vi "SYST_SHOR_PATH.vi"(0 "VISA IN":refnum<visa-resource-name>, 1 "Path":string, 5 "error in":errorcluster, 7 "Number":i32) -> (14 "VISA Out":refnum<visa-resource-name>, 19 "error out":errorcluster)   [LabVIEW 2018, in "PNA-X.lvlib"]
doc: "SYSTem:SHORtcut<n>:PATH <string> \n(Read-Write) Defines a Macro (shortcut) by linking a path and file name to the Macro number. To be \nexecuted, the executable file must be put in the PNA at the location indicated by this command. \nParameters \n<n> Numeric. Number of the macro to be stored in the analyzer. If the index \nnumber already exists, the existing macro is replaced with the new macro. \n<string> Full path, file name, and extension, of the existing macro \"executable\" file. \nTo find the number of a macro, either open the Macro Setup dialog and count \nthe line number of the desired macro, or query the titles of all 12 macros for the \ndesired macro title. \nExamples SYST:SHOR1:PATH \"C:\\Program Files\\Agilent\\Network \nAnalyzer\\Documents\\unguideMultiple.vbs\" \nQuery Syntax SYSTem:SHORtcut<n>:PATH? \nDefault Not Applicable"
uses:
  PNA-X.lvlib
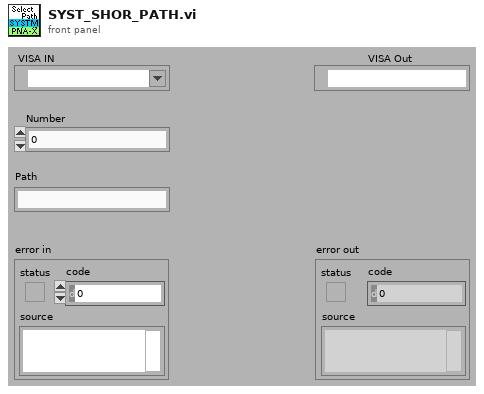
[diagram p1: front panel]
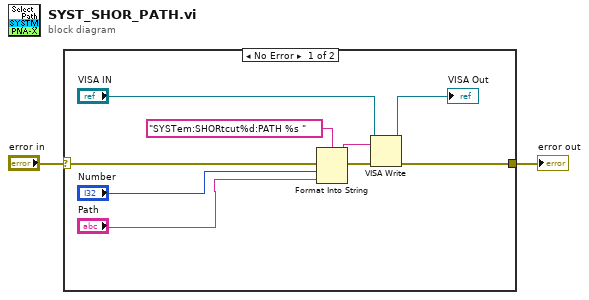
[diagram p0: block diagram]
diagram:
  n1 = case shown="No Error" "error in" {
    selector: "error in" -> [w11 w12]
    tunnel: [w6 w12] -> w1
    frame No Error {
      n2 = Format Into String(format string="SYSTem:SHORtcut%d:PATH %s " ("Cmdline"), error in=w11, "Number", "Path") -> (resulting string=w9:string, error out=w10:errorcluster)  [unwired: 1 in]
      n3 = VISA Write(VISA resource name="VISA IN", write buffer=w9, error in (no error)=w10) -> (VISA resource name out=→"VISA Out":refnum<visa-resource-name>, error out=w6:errorcluster)  [unwired: 1 out]
    }
    frame Error {
    }
  }
  "error out" <- w1
